vi "Move Until Limit.vi"(8 "error in (no error)":errorcluster, 10 "Speed":dbl, 11 "arm.lvclass":refnum<class "arm.lvclass">) -> (0 "error out":errorcluster, 3 "arm.lvclass":refnum<class "arm.lvclass">)   [LabVIEW 2015, in "arm.lvclass"]
uses:
  arm.lvclass
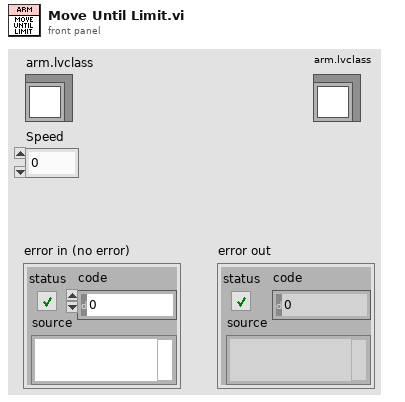
[diagram p1: front panel]
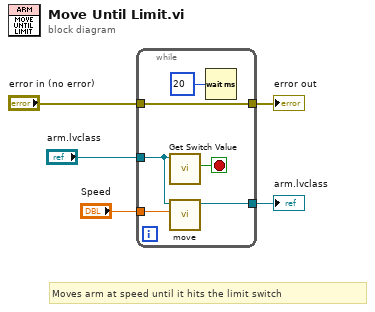
[diagram p0: block diagram]
diagram:
  # "Moves arm at speed until it hits the limit switch"
  n1 = while {
    tunnel: "arm.lvclass" -> [w6]
    tunnel: [w10] -> w3
    tunnel: "Speed" -> [w9]
    tunnel: "error in (no error)" -> [w8]
    tunnel: [w8] -> w1
    stop <- w7 stop-if-true
    n2 = call "Get Switch Value.vi"("arm.lvclass"=w6) -> ("Switch Pressed"=w7:bool)  [unwired: 9 in, 1 out]
    n3 = call "move.vi"("Speed"=w9, "arm.lvclass"=w6) -> ("arm.lvclass"=w10:refnum<class "arm.lvclass">)  [unwired: 9 in]
    n4 = Wait (ms)(milliseconds to wait=u32 20) -> ()  [unwired: 1 out]
  }
  "arm.lvclass" <- w3
  "error out" <- w1
